vi "SailSetSuggestions.vi"() -> ()   [LabVIEW 2012]
panel:
  in  "DesiredHeading":dbl
  in  "RobotHeading":dbl
  in  "RudderForce":dbl
  in  "DegreeOfLuffing":dbl
  in  "RelativeWindAngle":dbl
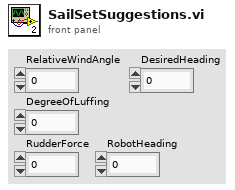
[diagram p1: front panel]
types:
  T1 = enum16{"Straight", "Turning", "Tacking", "Approach Maneuver", "Cross Wind (Tack)", "Cross Wind (Gybe)", "Turtle Mode", ""}
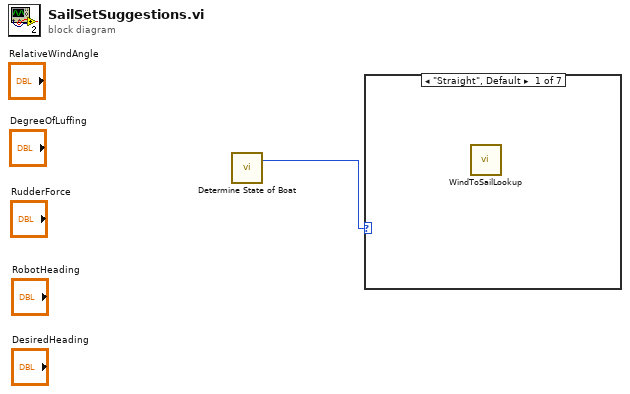
[diagram p0: block diagram]
diagram:
  n1 = call "Determine State of Boat.vi"() -> ("State of Boat"=w1:T1)  [unwired: 11 in]
  n2 = case shown="\"Straight\", Default" w1 {
    frame "Straight", Default {
      n3 = call "WindToSailLookup.vi"() -> ()  [unwired: 12 in]
    }
    frame "Turning" {
    }
    frame "Approach Maneuver" {
    }
    frame "Cross Wind (Tack)" {
    }
    frame "Cross Wind (Gybe)" {
    }
    frame "Turtle Mode" {
    }
    frame "Tacking" {
    }
  }
